vi "Caps Operator.vi"(0 "Data":T3, 1 "Data Cluster":T2, 2 "Physical Channel Index Cluster":T1, 5 "error in":errorcluster, 6 "Command":T13, 8 "Write a Register?":bool) -> (14 "Data 2":T3, 15 "Data Cluster 2":T2, 16 "Physical Channel Index Cluster 2":T1, 19 "error out":errorcluster)   [LabVIEW 2017]
uses:
  Ctrl/Property.ctl
  Ctrl/PhysicalChannel.ctl
  Ctrl/Bitfield.ctl
  Ctrl/Register.ctl
  Ctrl/ScaleType.ctl
  Ctrl/Scale.ctl
  Ctrl/EnumValue.ctl
  Ctrl/Enum.ctl
  Ctrl/Caps.ctl
  Ctrl/Data.ctl
  Ctrl/compond_2 commands.ctl
  Ctrl/User Input Cluster.ctl
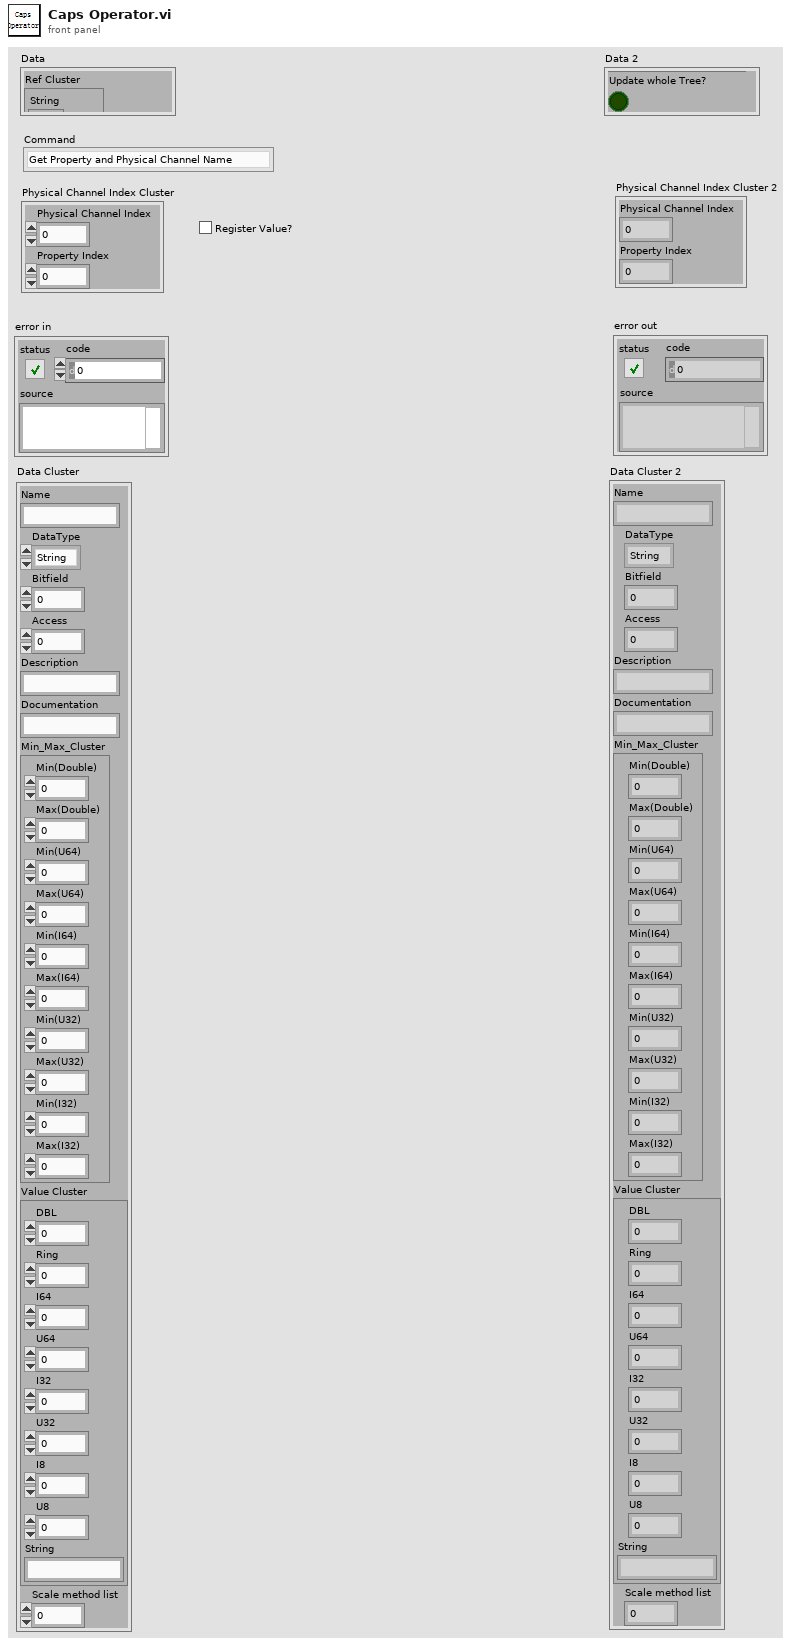
[diagram p1: front panel]
types:
  T1 = cluster{"Physical Channel Index":i32, "Property Index":i32}
  T2 = typedef "User Input Cluster.ctl" = cluster{"Name":string, "DataType":enum16{"String", "Double", "U64", "I64", "U32", "I32", "Bool"}, "Bitfield":u16, "Access":u16, "Description":string, "Documentation":string, "Min_Max_Cluster":cluster{"Min(Double)":dbl, "Max(Double)":dbl, "Min(U64)":u64, "Max(U64)":u64, "Min(I64)":i64, "Max(I64)":i64, "Min(U32)":u32, "Max(U32)":u32, "Min(I32)":i32, "Max(I32)":i32}, "Value Cluster":cluster{"DBL":dbl, "Ring":u16, "I64":i64, "U64":u64, "I32":i32, "U32":u32, "I8":i8, "U8":u8, "String":string}, "Scale method list":u16}
  T3 = typedef "Data.ctl" = cluster{"Ref Cluster":cluster{"String":refnum<vi>, "U8":refnum<vi>, "I8":refnum<vi>, "U32":refnum<vi>, "I32":refnum<vi>, "U64":refnum<vi>, "I64":refnum<vi>, "Ring":refnum<vi>, "DBL":refnum<vi>, "Add":refnum<vi>, "Remove":refnum<vi>, "Property tree":refnum<vi>}, "JSON Text":string, "Original JSON Text":string, "Caps":T4, "SLSC Output Tree":cluster{"Left Cell String":string, "Child Text":string[], "Child Tag":string, "Item Indent":i32, "Child Only?":bool, "Glyph Index":i32, "offline value":variant}[], "Ref Index and Control Type":cluster{"index":i32, "Datatype":string}, "Selected Type and name":cluster{"Selected Type":enum16{"Property", "Physical Channel"}, "Selected Property Name":string}, "Update whole Tree?":bool}
  T4 = typedef "Caps.ctl" = cluster{"properties":T5[], "physical channels":T6[], "registers":T7[], "scales":T9[], "enums":T11[], "productName":string}
  T5 = typedef "Property.ctl" = cluster{"name":string, "bitfield":string, "value":variant, "dataType":string, "min":variant, "max":variant, "scale":string, "access":string}
  T6 = typedef "PhysicalChannel.ctl" = cluster{"name":string, "properties":T5[]}
  T7 = typedef "Register.ctl" = cluster{"name":string, "address":i32, "size":i32, "bitfields":T8[], "initialValue":variant, "connectedProperties":string[]}
  T8 = typedef "Bitfield.ctl" = cluster{"name":string, "offset":i32, "size":i32, "signed":bool}
  T9 = typedef "Scale.ctl" = cluster{"name":string, "type":T10, "params":variant}
  T10 = typedef "ScaleType.ctl" = enum16{"NoScale", "Table", "Polynomial", "Linear"}
  T11 = typedef "Enum.ctl" = cluster{"name":string, "values":T12[]}
  T12 = typedef "EnumValue.ctl" = cluster{"name":string, "value":i32}
  T13 = typedef "compond_2 commands.ctl" = enum16{"Get Property and Physical Channel Name", "Get the Type and Value", "Add new Value", "Modify the Value"}
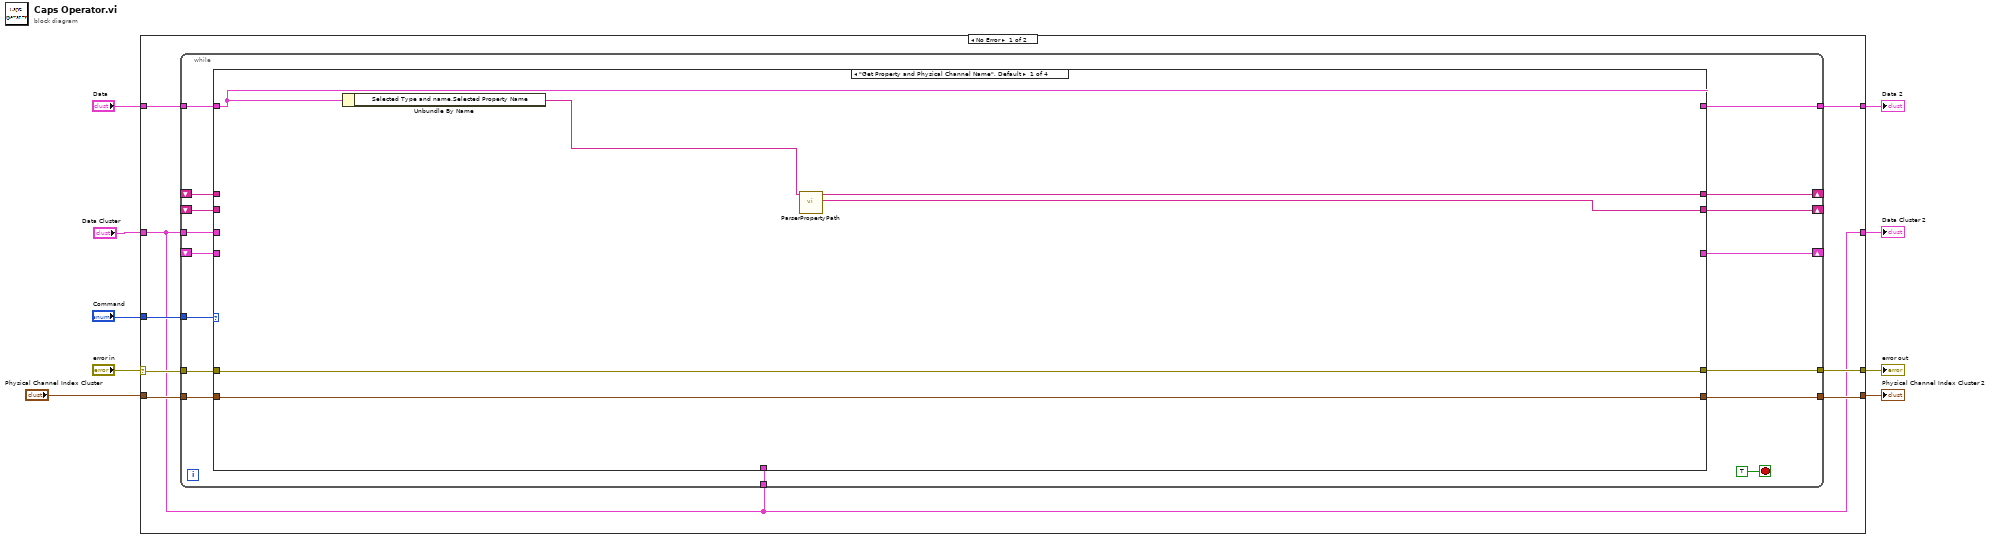
[diagram p0: block diagram]
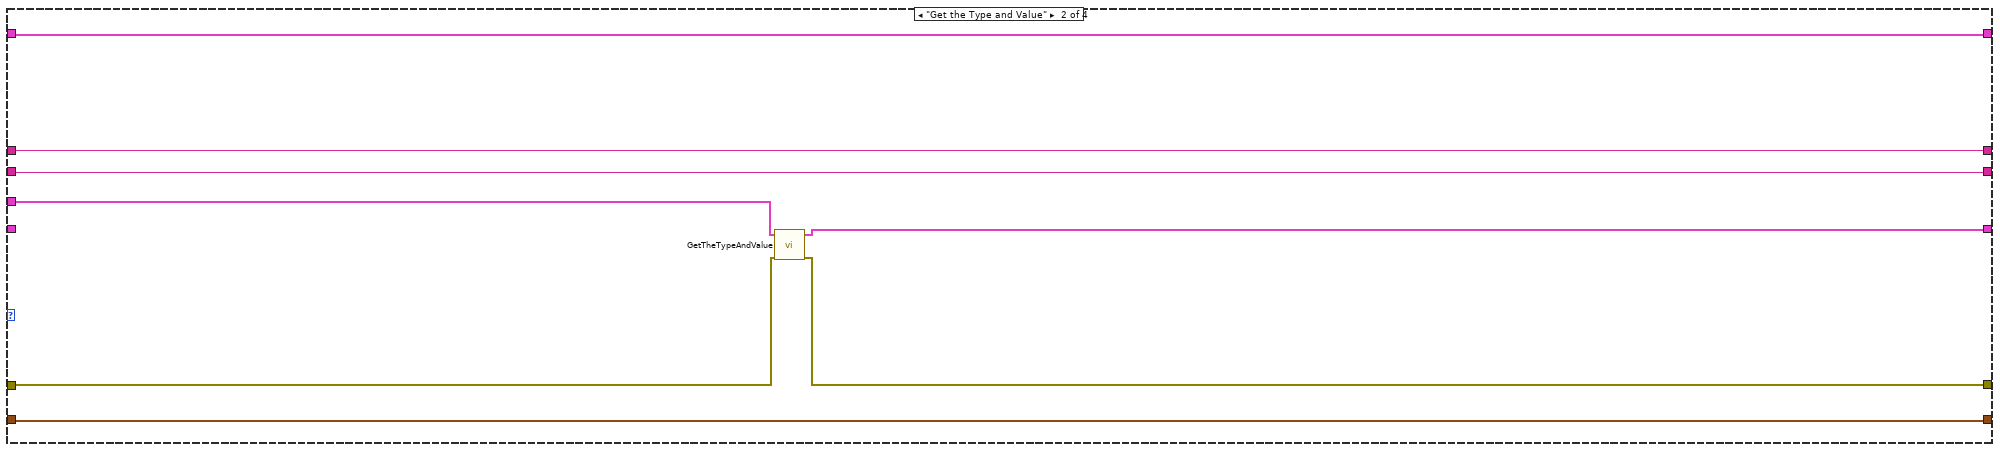
[diagram p2: hidden frame]
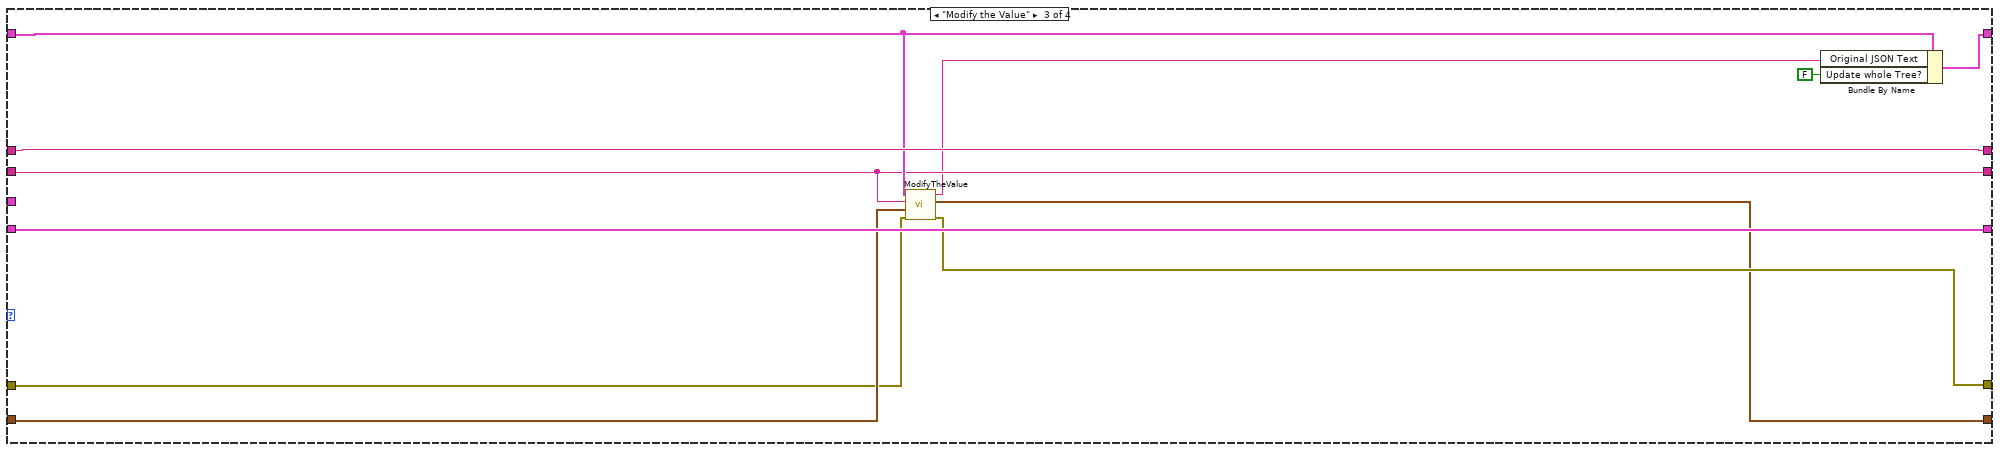
[diagram p3: hidden frame]
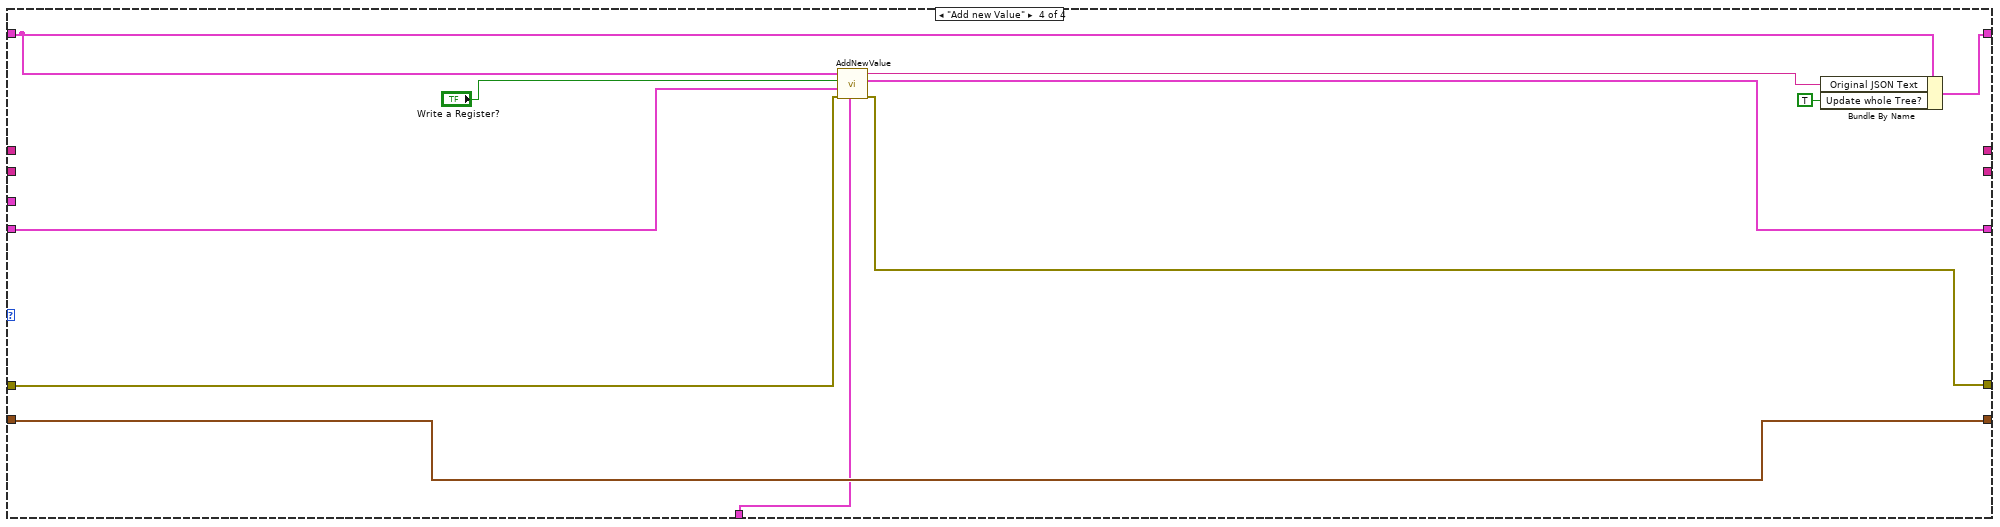
[diagram p4: hidden frame]
diagram:
  n1 = case shown="No Error" "error in" {
    selector: "error in" -> [w15 w72]
    tunnel: "Data" -> [w17 w73]
    tunnel: "Command" -> [w16 _]
    tunnel: [w14 w73] -> w7
    tunnel: "Data Cluster" -> [w10 w71]
    tunnel: [w13 w72] -> w5
    tunnel: [w10 w71] -> w4
    tunnel: "Physical Channel Index Cluster" -> [w12 w70]
    tunnel: [w11 w70] -> w2
    frame No Error {
      n2 = while {
        tunnel: w17 -> [w32]
        tunnel: w16 -> [w31]
        tunnel: w15 -> [w30]
        shift-right: [w29] -> _
        shift-left: _ -> [w27]
        shift-right: [w28] -> _
        shift-left: _ -> [w26]
        tunnel: [w18] -> w14
        tunnel: w10 -> [w25]
        shift-right: [w24] -> _
        shift-left: _ -> [w23]
        tunnel: [w22] -> w13
        tunnel: w12 -> [w21]
        tunnel: [w20] -> w11
        tunnel: w10 -> [w19]
        stop <- TRUE stop-if-true
        n3 = case shown="\"Get Property and Physical Channel Name\", Default" w31 {
          tunnel: w32 -> [w39 w47 w54 w66]
          tunnel: w30 -> [w38 w41 w51 w63]
          tunnel: [w35 w46 w56 _] -> w29
          tunnel: [w34 w45 w53 _] -> w28
          tunnel: w27 -> [_ w46 w56 _]
          tunnel: w26 -> [_ w45 w53 _]
          tunnel: [w39 w47 w58 w69] -> w18
          tunnel: w25 -> [_ w43 _ _]
          tunnel: [_ w42 w57 w60] -> w24
          tunnel: w23 -> [_ _ w57 w64]
          tunnel: [w38 w40 w50 w59] -> w22
          tunnel: w21 -> [w37 w44 w52 w68]
          tunnel: [w37 w44 w49 w68] -> w20
          tunnel: w19 -> [_ _ _ w62]
          frame "Get Property and Physical Channel Name", Default {
            n4 = Unbundle By Name(w39) -> ("Selected Type and name.Selected Property Name"=w36:string)
            n5 = call "ParserPropertyPath.vi"("property"=w36) -> ("name"=w34:string, "pyhsical channel"=w35:string)  [unwired: 7 in]
          }
          frame "Get the Type and Value" {
            n6 = call "GetTheTypeAndValue.vi"("error in (no error)"=w41, "Data Cluster"=w43) -> ("error out"=w40:errorcluster, "DataType and Value"=w42:cluster{"Type":string, "Value":variant})  [unwired: 8 in]
          }
          frame "Modify the Value" {
            n7 = call "ModifyTheValue.vi"("error in (no error)"=w51, "Physical Channel Index Cluster"=w52, "name"=w53, "Data"=w54) -> ("error out"=w50:errorcluster, "Physical Channel Index Cluster Out"=w49:T1, "JSON Text Out"=w48:string)  [unwired: 5 in]
            n8 = Bundle By Name(cluster=w54, "Original JSON Text"=w48, "Update whole Tree?"=FALSE) -> (w58:T3)
          }
          frame "Add new Value" {
            n9 = call "AddNewValue.vi"("Data Cluster"=w62, "error IO"=w63, "DataType and Value"=w64, "Write a Register?"="Write a Register?", "Data"=w66) -> ("error IO Out"=w59:errorcluster, "DataType and Value Out"=w60:cluster{"Type":string, "Value":variant}, "JSON Text Out"=w61:string)  [unwired: 4 in]
            n10 = Bundle By Name(cluster=w66, "Original JSON Text"=w61, "Update whole Tree?"=TRUE) -> (w69:T3)
          }
        }
      }
    }
    frame Error {
    }
  }
  "error out" <- w5
  "Data 2" <- w7
  "Data Cluster 2" <- w4
  "Physical Channel Index Cluster 2" <- w2
